vi "Y-1D-temp.vi"(3 "row in":sgl[](array[numeric]), 4 "array in":sgl[](array[numeric]), 5 "command":enum16{"get", "set", "clear", "append"}(ring)) -> (0 "range":cluster{"min":sgl, "max":sgl}, 1 "array out":sgl[](array[numeric]))   [LabVIEW 2013]
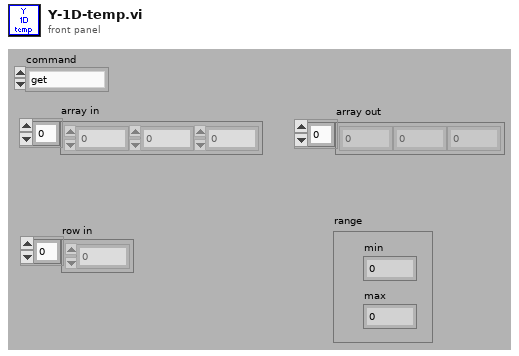
[diagram p1: front panel]
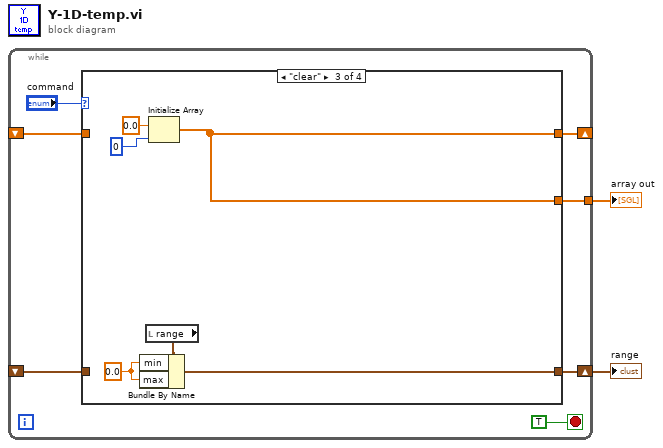
[diagram p0: block diagram]
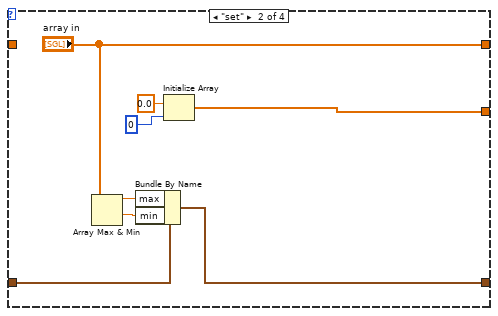
[diagram p3: hidden frame]
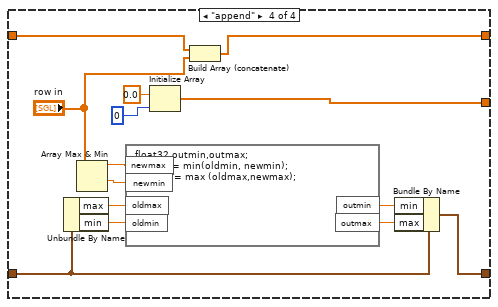
[diagram p4: hidden frame]
diagram:
  n1 = while {
    shift-right: [w7] -> _
    shift-left: _ -> [w8]
    tunnel: [w6] -> w2
    shift-right: [w5] -> w1
    shift-left: _ -> [w4]
    stop <- TRUE stop-if-true
    n2 = case shown="\"clear\"" "command" {
      tunnel: [w11 "array in" w23 w27] -> w7
      tunnel: w8 -> [w11 _ _ w26]
      tunnel: [w11 w17 w23 w37] -> w6
      tunnel: [w10 w12 w20 w29] -> w5
      tunnel: w4 -> [w10 w13 _ w30]
      frame "get", Default {
      }
      frame "set" {
        n3 = Array Max & Min(array="array in") -> (max value=w15:sgl, min value=w14:sgl)  [unwired: 2 out]
        n4 = Bundle By Name(cluster=w13, "max"=w15, "min"=w14) -> (w12:cluster{"min":sgl, "max":sgl})
        n5 = Initialize Array(sgl 0.0 ("element"), 0 ("dimension size")) -> (w17:sgl[])
      }
      frame "clear" {
        w21 = sgl 0.0 ("min")
        n6 = local read "range"() -> (w22:cluster{"min":sgl, "max":sgl})
        n7 = Bundle By Name(cluster=w22, "min"=w21, "max"=w21) -> (w20:cluster{"min":sgl, "max":sgl})
        n8 = Initialize Array(sgl 0.0 ("element"), 0 ("dimension size")) -> (w23:sgl[])
      }
      frame "append" {
        n9 = Unbundle By Name(w30) -> ("max"=w34:sgl, "min"=w33:sgl)
        n10 = Array Max & Min(array="row in") -> (max value=w36:sgl, min value=w35:sgl)  [unwired: 2 out]
        n11 = formula code="float32 outmin,outmax;\noutmin = min(oldmin, newmin);\noutmax = max (oldmax,newmax);"("oldmin"=w33, "oldmax"=w34, "newmax"=w36, "newmin"=w35) -> ("outmin"=w32:sgl, "outmax"=w31:sgl)
        n12 = Initialize Array(sgl 0.0 ("element"), 0 ("dimension size")) -> (w37:sgl[])
        n13 = Build Array (concatenate)(w26, "row in") -> (w27:sgl[])
        n14 = Bundle By Name(cluster=w30, "min"=w32, "max"=w31) -> (w29:cluster{"min":sgl, "max":sgl})
      }
    }
  }
  "array out" <- w2
  "range" <- w1
